vi "Actor Core Dups.vi"(8 "error in":errorcluster, 11 "Stepper3D in":refnum<class "Stepper3D.lvclass">) -> (0 "error out":errorcluster, 3 "Actor  out":refnum<class "Actor.lvclass">)   [LabVIEW 2014]
uses:
  <vilib>/Utility/config.llb/NI_LVConfig.lvlib
  <vilib>/Utility/error.llb/DialogType.ctl
  Libs/array.lib/Array.lvlib
  Libs/stepper3D.lib/stepper3D.lvlib
  Libs/stepper3D.lib/Enums/BoundaryStatus.ctl
  <vilib>/Utility/config.llb/Read Key (Double).vi
  <vilib>/Utility/config.llb/Write Key (Double).vi
  Framework/Interfaces/Viewable Actor/Viewable Actor.lvclass
  Framework/Interfaces/Observable Actor/Observable Actor.lvclass
  Framework/Model/Data/DataSingleElement/DataSingleElement.lvclass
  Framework/Hardware/ParameterDevice/ParameterDevice Messages/Set Parameter Msg/Set Parameter Msg.lvclass
  <vilib>/ActorFramework/Actor/Actor.lvclass
  Stepper3D Messages/Set Conversion Table Msg/Set Conversion Table Msg.lvclass
  Libs/stepper3D.lib/Enums/CurrentStatus.ctl
  Stepper3D Messages/Refresh Info Msg/Refresh Info Msg.lvclass
  Framework/Hardware/Device/Device Messages/Connect Msg/Connect Msg.lvclass
  Framework/Hardware/Device/Device Messages/Disconnect Msg/Disconnect Msg.lvclass
  Stepper3D.lvclass
panel:
  out "WL:Real Value":dbl=450.0
  out "Stop":bool=TRUE
  out "St3:Right":bool
  out "St3:Left":bool
  out "St2:Right":bool
  out "St2:Left":bool
  out "St1:Right":bool
  out "St1:Left":bool
  in  "Speed":string="300"
  in  "UI:LoadConversionTables":bool
  in  "Conversion 3":path=path "C:/Users/219-PC/Dropbox/МФД/Alexandr Bogomolov/Кумарин 47/Эталон.txt"
  in  "Conversion 2":path=path "C:/Users/219-PC/Dropbox/МФД/Alexandr Bogomolov/Кумарин 47/Эталон.txt"
  in  "Conversion 1":path=path "C:/Users/219-PC/Dropbox/МФД/Alexandr Bogomolov/Кумарин 47/Решетка 3D.txt"
  out "WL:WLToStepper3":dbl[][](array[numeric])
  out "WL:WLToStepper2":dbl[][](array[numeric])=[[115.0, 0.0], [135.0, 0.0]]
  out "WL:WLToStepper1":dbl[][](array[numeric])
  in  "WL:NewValue":dbl=450.0
  in  "WL:Stop":bool
  in  "WL:SetValue":bool
  out "App:RefreshLED":bool
  in  "App:RefreshRate":u32=500 caption="Refresh every"
  in  "App:Refresh":bool
  in  "App:Disconnect":bool
  in  "App:Connect":bool
  in  "St3:SetPos":bool
  in  "St2:SetPos":bool
  in  "St1:SetPos":bool
  in  "St:Stop":bool
  in  "St3:Steps":dbl
  in  "St3:NewPosition":dbl=2605.0
  out "St3:Position":dbl=2903.0
  in  "St2:Steps":dbl
  in  "St2:NewPosition":dbl=-2500.0
  out "St2:Position":dbl=-2500.0
  in  "St:DoSteps":bool
  in  "St1:Steps":dbl
  in  "St1:NewPosition":dbl=-57680.0
  out "St1:Position":dbl=-57680.0
  in  "App:ResourceName":refnum<visa-resource-name>="COM8"
  # "ms."
  # "BOUNDARY"
  # "FUNCTIONS"
  # "POSITION"
  # "NEW POSITION"
  # "STEPS"
  # "Решетка"
  # "Фабри-Перо"
  # "Кристалл"
  # "Длина волны"
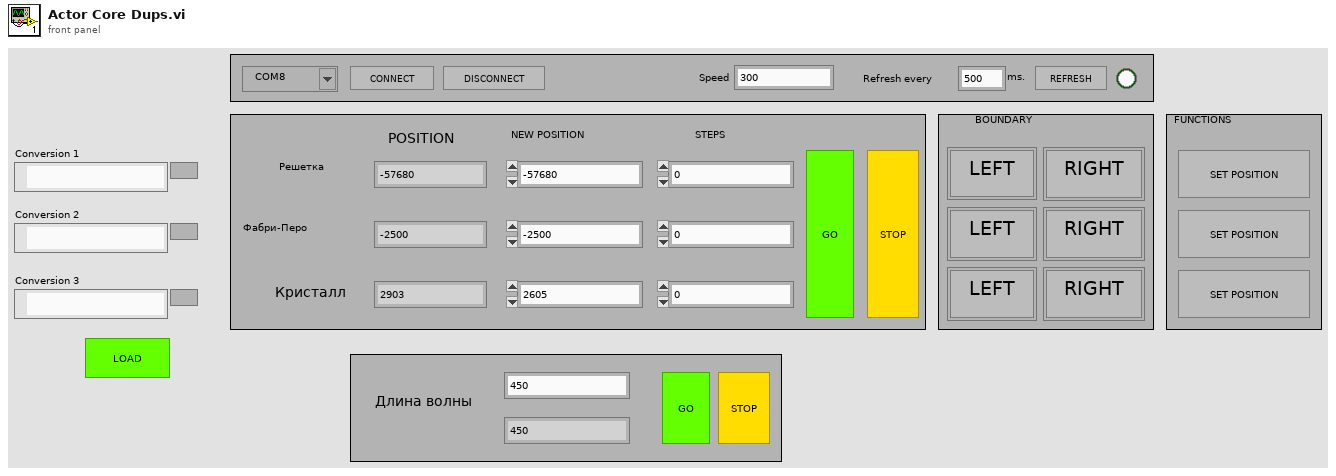
[diagram p1: front panel]
types:
  T1 = typedef "Observable Actor.lvlib/Observable Actor.lvclass/Observer.ctl" = refnum<queue>
  T2 = typedef "stepper3D.lvlib/CurrentStatus.ctl" = cluster{"desired":dbl[], "current":dbl[], "boundaries":T3[], "is running":bool}
  T3 = typedef "stepper3D.lvlib/BoundaryStatus.ctl" = enum16{"NO BOUNDARY", "OUT OF LEFT", "OUT OF RIGHT"}
  T4 = enum32{"invalid app kind", "Development System", "Run Time System", "Student Edition", "Embedded LabVIEW", "Evaluation", "Custom"}
  T5 = cluster{"Core":cluster{"Current VI Reference":refnum<vi>, "Close Panel on Exit?":bool}, "App:RefreshRate":u32, "appended path":path, "App:ResourceName":refnum<visa-resource-name>}
  T6 = typedef "DialogType.ctl" = u16
  T7 = cluster{"Current VI Reference":refnum<vi>, "Close Panel on Exit?":bool}
  T8 = typedef "NI_LVConfig.lvlib/Config Data RefNum.ctl" = refnum<k1>
  T9 = enum8{"Enabled", "Disabled", "Disabled and Grayed Out"}
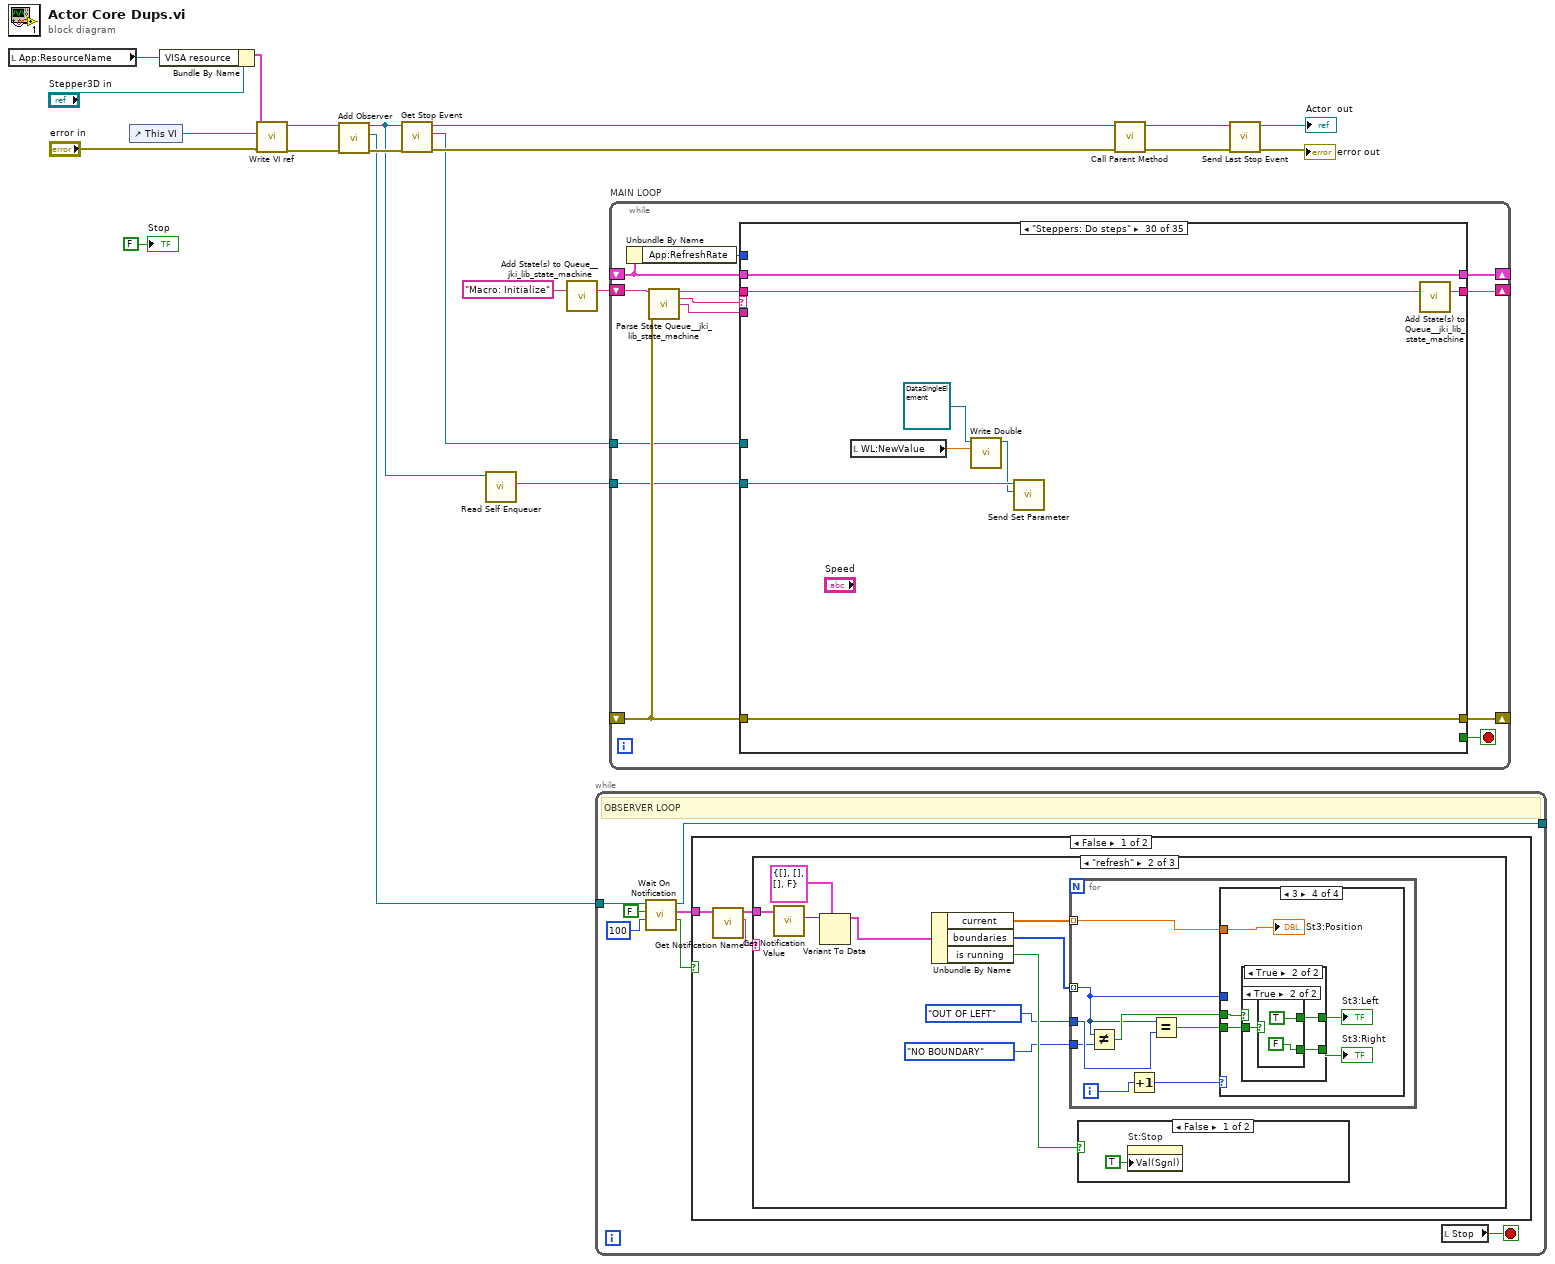
[diagram p0: block diagram]
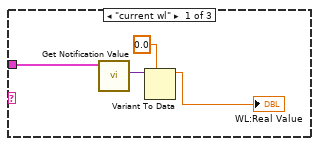
[diagram p2: hidden frame]
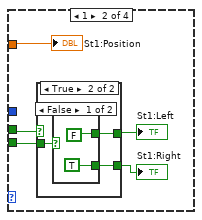
[diagram p5: hidden frame]
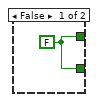
[diagram p6: hidden frame]
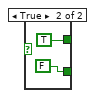
[diagram p7: hidden frame]
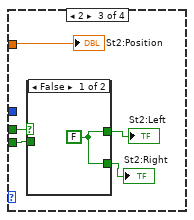
[diagram p8: hidden frame]
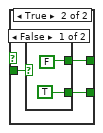
[diagram p9: hidden frame]
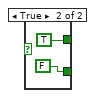
[diagram p10: hidden frame]
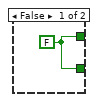
[diagram p11: hidden frame]
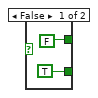
[diagram p12: hidden frame]
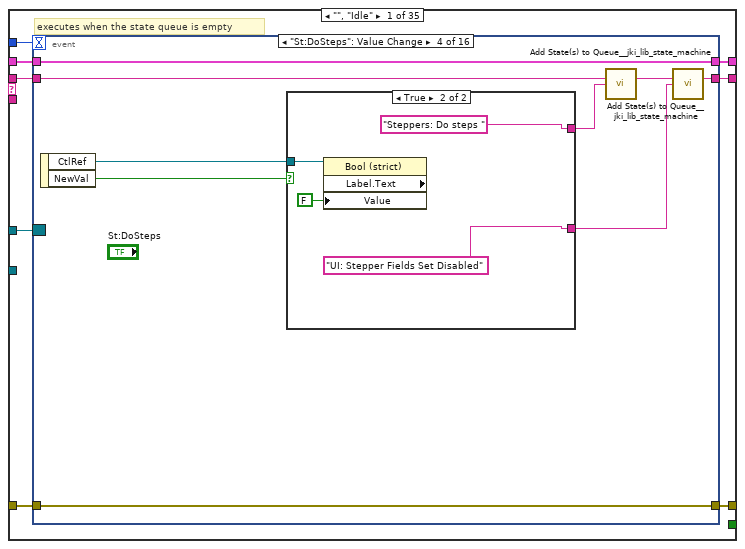
[diagram p15: hidden frame]
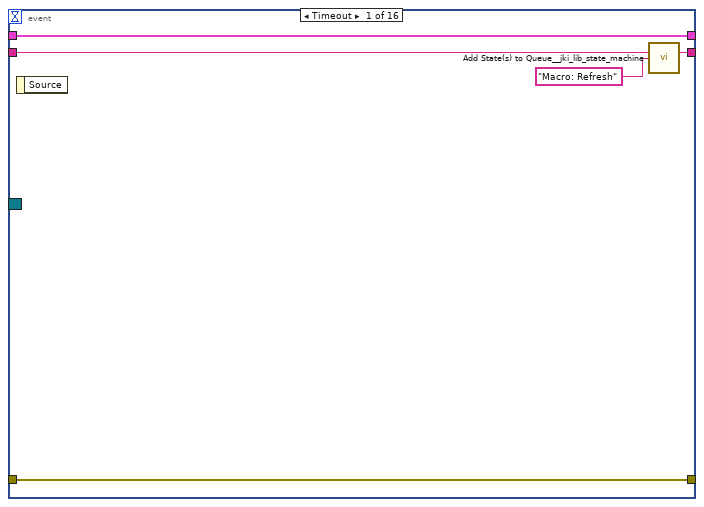
[diagram p16: hidden frame]
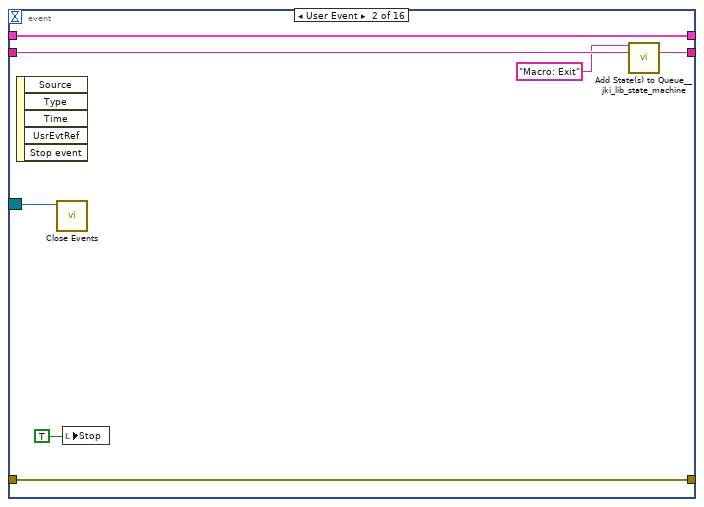
[diagram p17: hidden frame]
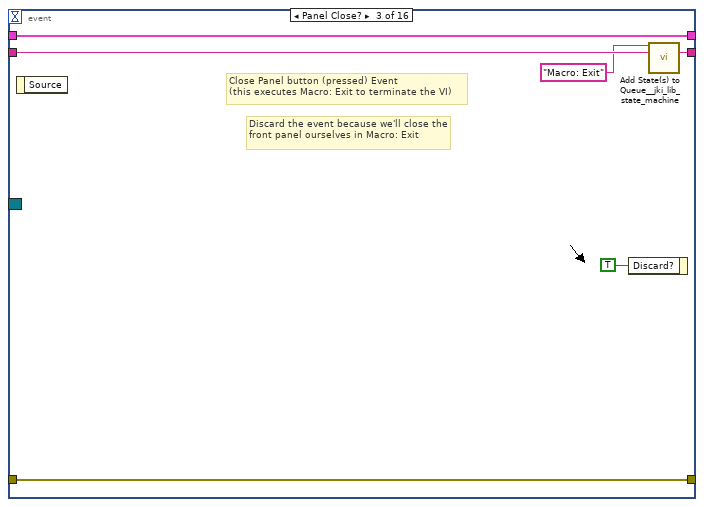
[diagram p18: hidden frame]
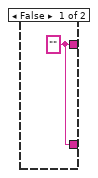
[diagram p19: hidden frame]
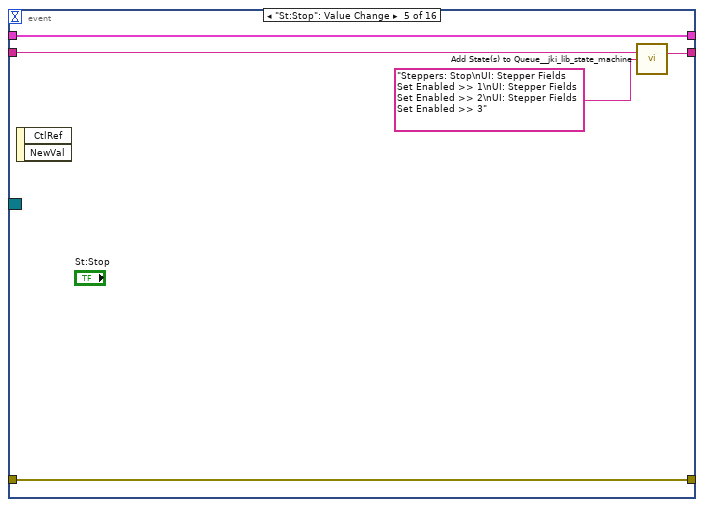
[diagram p20: hidden frame]
diagram:
  n1 = local read "App:ResourceName"() -> (w1:refnum<visa-resource-name>)
  n2 = control-ref of="This VI"() -> (w16:refnum<vi>)
  n3 = Bundle By Name(cluster="Stepper3D in", "VISA resource"=w1) -> (w3:cluster{})
  n4 = call "Write VI ref.vi"("error in (no error)"="error in", "VI ref"=w16, "Viewable Actor in"=w3) -> ("error out"=w18:errorcluster, "Viewable Actor out"=w17:refnum<class "Viewable Actor.lvclass">)  [unwired: 7 in]
  n5 = call-dynamic "Add Observer.vi"("error in (no error)"=w18, "Observable Actor in"=w17) -> ("error out"=w19:errorcluster, "new observer"=w6:T1, "Observable Actor out"=w5:refnum<class "Viewable Actor.lvclass">)  [unwired: 7 in]
  n6 = call-dynamic "Get Stop Event.vi"("error in (no error)"=w19, "Observable Actor in"=w5) -> ("error out"=w10:errorcluster, "Events"=w7:refnum<event-registration>, "Observable Actor out"=w11:refnum<class "Viewable Actor.lvclass">)  [unwired: 7 in]
  n7 = call <vilib>:"Read Self Enqueuer.vi"("Actor"=w5) -> ("Self Enqueuer"=w4:refnum<class "Message Enqueuer.lvclass">)  [unwired: 10 in]
  n8 = call <vilib>:"Add State(s) to Queue__jki_lib_state_machine.vi"("State(s) in (\"\")"="Macro: Initialize") -> ("States Out"=w21:string)  [unwired: 14 in]
  n9 = while {
    tunnel: w6 -> [w26]
    tunnel: [w25] -> _
    stop <- w22 stop-if-true
    # "OBSERVER LOOP"
    n10 = call "Wait On Notification.vi"("timeout in ms (-1)"=100, "ignore previous (F)"=FALSE, "observer in"=w26) -> ("timed out?"=w23:bool, "notification"=w24:cluster{"value":variant, "name":string}, "observer out"=w25:T1)  [unwired: 5 in, 1 out]
    n11 = case shown="False" w23 {
      tunnel: w24 -> [w31 _]
      frame False {
        n12 = call "Get Notification Name.vi"("notification in"=w31) -> ("name"=w29:string, "notification out"=w30:cluster{"value":variant, "name":string})  [unwired: 9 in]
        n13 = case shown="\"refresh\"" w29 {
          tunnel: w30 -> [w33 w43 _]
          frame "current wl" {
            n14 = call "Get Notification Value.vi"("notification in"=w33) -> ("data"=w35:variant)  [unwired: 7 in, 1 out]
            n15 = Variant To Data(type=0.0 ("Current value"), Variant=w35) -> (data=→"WL:Real Value":dbl)  [unwired: 1 in, 1 out]
          }
          frame "refresh" {
            n16 = call "Get Notification Value.vi"("notification in"=w43) -> ("data"=w44:variant)  [unwired: 7 in, 1 out]
            n17 = Variant To Data(type=T2 {"desired"=[], "current"=[], "boundaries"=[], "is running"=FALSE} ("status"), Variant=w44) -> (data=w37:T2)  [unwired: 1 in, 1 out]
            n18 = Unbundle By Name(w37) -> ("current"=w38:dbl[], "boundaries"=w39:T3[], "is running"=w42:bool)
            n19 = for {
              tunnel: w38 -> [w51] mode=indexing
              tunnel: w39 -> [w48] mode=indexing
              tunnel: BoundaryStatus."NO BOUNDARY" ("Enum") -> [w46]
              tunnel: BoundaryStatus."OUT OF LEFT" ("Enum") -> [w49]
              i -> [w53]
              n20 = Not Equal?(x=w48, y=w46) -> (x != y?=w50:bool)
              n21 = Increment(x=w53) -> (x+1=w52:i32)
              n22 = Equal?(x=w48, y=w49) -> (x = y?=w47:bool)
              n23 = case shown="3" w52 {
                tunnel: w51 -> [_ w58 w71 w84]
                tunnel: w48 -> [_ _ _ _]
                tunnel: w50 -> [_ w57 w70 w83]
                tunnel: w47 -> [_ w56 w69 w82]
                frame Default {
                }
                frame 1 {
                  n24 = case shown="True" w57 {
                    tunnel: w56 -> [_ w62]
                    tunnel: [w59 w61] -> w55
                    tunnel: [w59 w60] -> w54
                    frame False {
                      w59 = FALSE
                    }
                    frame True {
                      n25 = case shown="False" w62 {
                        tunnel: [FALSE TRUE] -> w61
                        tunnel: [TRUE FALSE] -> w60
                        frame False {
                        }
                        frame True {
                        }
                      }
                    }
                  }
                  "St1:Right" <- w54
                  "St1:Left" <- w55
                  "St1:Position" <- w58
                }
                frame 2 {
                  n26 = case shown="False" w70 {
                    tunnel: w69 -> [_ w75]
                    tunnel: [w72 w74] -> w68
                    tunnel: [w72 w73] -> w67
                    frame False {
                      w72 = FALSE
                    }
                    frame True {
                      n27 = case shown="False" w75 {
                        tunnel: [FALSE TRUE] -> w74
                        tunnel: [TRUE FALSE] -> w73
                        frame False {
                        }
                        frame True {
                        }
                      }
                    }
                  }
                  "St2:Left" <- w68
                  "St2:Right" <- w67
                  "St2:Position" <- w71
                }
                frame 3 {
                  n28 = case shown="True" w83 {
                    tunnel: w82 -> [_ w88]
                    tunnel: [w85 w87] -> w80
                    tunnel: [w85 w86] -> w81
                    frame False {
                      w85 = FALSE
                    }
                    frame True {
                      n29 = case shown="True" w88 {
                        tunnel: [FALSE TRUE] -> w87
                        tunnel: [TRUE FALSE] -> w86
                        frame False {
                        }
                        frame True {
                        }
                      }
                    }
                  }
                  "St3:Left" <- w80
                  "St3:Right" <- w81
                  "St3:Position" <- w84
                }
              }
            }
            n30 = case shown="False" w42 {
              frame False {
                n31 = property on="St:Stop" class="Bool (strict)"("Val(Sgnl)"=TRUE) -> ()  [unwired: 2 in, 2 out]
              }
              frame True {
              }
            }
          }
          frame Default {
          }
        }
      }
      frame True {
      }
    }
    n32 = local read "Stop"() -> (w22:bool)
  }
  n33 = while "MAIN LOOP" {
    shift-right: [w99] -> _
    shift-left: _ -> [w95]
    shift-right: [w102] -> _
    shift-left: _ -> [w98]
    shift-right: [w101] -> _
    shift-left: w21 -> [w103]
    tunnel: w7 -> [w94]
    tunnel: w4 -> [w93]
    stop <- w100 stop-if-true
    n34 = Unbundle By Name(w95) -> ("App:RefreshRate"=w96:u32)
    n35 = call <vilib>:"Parse State Queue__jki_lib_state_machine.vi"("State Queue"=w103, "Error In (no error)"=w98) -> ("Remaining States"=w105:string, "Current State"=w97:string, "Arguments"=w104:string)  [unwired: 11 in]
    n36 = case shown="\"Steppers: Do steps\"" w97 {
      selector: w97 -> [_ _ w260 _ _ _ _ _ _ _ _ _ _ _ _ _ _ _ _ _ _ _ _ _ _ _ _ _ _ _ _ _ _ _ _]
      tunnel: w105 -> [w113 w259 w264 w282 w289 w294 w298 w315 w325 w344 w366 w372 w376 w381 w386 w391 w393 w412 w415 w431 w432 w439 w454 w459 w464 w474 w478 w484 w490 w498 w513 w524 w530 w535 w542]
      tunnel: w104 -> [_ _ _ _ _ _ _ _ _ _ _ _ _ _ _ _ w392 _ w416 _ w435 w440 _ _ _ _ _ _ _ _ w509 _ _ _ w538]
      tunnel: w95 -> [w111 w256 w262 w273 w286 w292 w295 w312 _ w342 w363 w368 w373 w378 w383 w389 w395 w414 w418 w429 w436 w442 w451 w456 w461 w471 w475 w480 w486 w496 w510 w522 w531 w532 w539]
      tunnel: [w110 w257 w266 w279 errorcluster {"status"=FALSE, "code"=0, "source"=""} ("error out") w291 w296 w313 w322 w326 w364 w369 w374 w379 w384 w388 w394 w413 w417 w428 w434 w443 w452 w457 w462 w472 w476 w479 w487 w495 w508 w519 w525 w533 w540] -> w102
      tunnel: w98 -> [w109 w257 w265 w279 w285 w291 w296 w313 w322 w327 w364 w367 w374 w379 w384 w388 w394 w413 w417 w428 w434 w444 w452 w457 w462 w472 w476 w481 w488 w495 w507 w520 w526 w533 w540]
      tunnel: [w112 w258 w263 w281 w288 w293 w297 w314 w324 w343 w365 w371 w375 w380 w385 w390 w393 w412 w415 w430 w432 w439 w453 w458 w463 w473 w477 w485 w490 w497 w512 w523 w529 w534 w541] -> w101
      tunnel: [_ _ _ _ _ TRUE _ _ _ _ _ _ _ _ _ _ _ _ _ _ _ _ _ _ _ _ _ _ _ _ _ _ _ _ _] -> w100
      tunnel: [w108 w256 w262 w280 w286 w292 w295 w312 w323 w342 w363 w368 w373 w378 w383 w389 w395 w414 w418 w429 w436 w442 w451 w456 w461 w471 w475 w480 w486 w496 w510 w522 w531 w532 w539] -> w99
      tunnel: w96 -> [w107 _ _ _ _ _ _ _ _ _ _ _ _ _ _ _ _ _ _ _ _ _ _ _ _ _ _ _ _ _ _ _ _ _ _]
      tunnel: w94 -> [w106 _ _ _ _ _ _ _ _ _ _ _ _ _ _ _ _ _ _ _ _ _ _ _ _ _ _ _ _ _ _ _ _ _ _]
      tunnel: w93 -> [_ _ _ _ _ _ _ w305 _ _ _ _ _ _ _ _ _ _ _ _ _ _ _ _ _ _ _ w482 w489 w494 _ _ w527 _ _]
      frame "", "Idle" {
        # "executes when the state queue is empty"
        n37 = event shown="[3] \"St:DoSteps\": Value Change" {
          selector: w106 -> [_ w121 _ _ _ _ _ _ _ _ _ _ _ _ _ _]
          dyn-events: _ -> [_ _ _ _ _ _ _ _ _ _ _ _ _ _ _ _]
          timeout: w107 -> [_ _ _ _ _ _ _ _ _ _ _ _ _ _ _ _]
          tunnel: w113 -> [w118 w122 w131 w136 w147 w153 w174 w185 w192 w202 w213 w227 w232 w237 w244 w252]
          tunnel: [w117 w123 w130 w134 w148 w152 w173 w184 w193 w203 w214 w228 w233 w238 w245 w253] -> w112
          tunnel: w111 -> [w115 w124 w128 w139 w150 w156 w176 w187 w194 w206 w217 w224 w230 w235 w242 w250]
          tunnel: [w116 w119 w129 w138 w149 w155 w175 w186 w195 w200 w211 w225 w231 w236 w243 w251] -> w110
          tunnel: w109 -> [w116 w119 w129 w138 w149 w155 w175 w186 w195 w200 w211 w225 w231 w236 w243 w251]
          tunnel: [w115 w124 w128 w139 w150 w156 w176 w187 w194 w206 w217 w223 w230 w235 w242 w250] -> w108
          event Timeout {
            n38 = event-data() -> ()  [unwired: 1 in, 1 out]
            n39 = call <vilib>:"Add State(s) to Queue__jki_lib_state_machine.vi"("State(s) in (\"\")"=w118, "State(s) at Back (\"\")"="Macro: Refresh") -> ("States Out"=w117:string)  [unwired: 13 in]
          }
          event User Event {
            n40 = event-data() -> ()  [unwired: 1 in, 5 out]
            n41 = call "Close Events.vi"("events"=w121) -> ()  [unwired: 11 in]
            n42 = local write "Stop"(TRUE) -> ()
            n43 = call <vilib>:"Add State(s) to Queue__jki_lib_state_machine.vi"("State(s) in Front (\"\")"="Macro: Exit", "State(s) in (\"\")"=w122) -> ("States Out"=w123:string)  [unwired: 13 in]
          }
          event Panel Close? {
            # "Discard the event because we'll close the front panel ourselves in Macro: Exit"
            # "Close Panel button (pressed) Event\n(this executes Macro: Exit to terminate the VI)"
            n44 = event-data() -> ()  [unwired: 1 in, 1 out]
            n45 = event-data("Discard?"=TRUE) -> ()  [unwired: 1 in, 1 out]
            n46 = call <vilib>:"Add State(s) to Queue__jki_lib_state_machine.vi"("State(s) in Front (\"\")"="Macro: Exit", "State(s) in (\"\")"=w131) -> ("States Out"=w130:string)  [unwired: 13 in]
          }
          event "St:DoSteps": Value Change {
            n47 = event-data() -> ("CtlRef"=w140:refnum<vi>, "NewVal"=w137:bool)  [unwired: 1 in]
            n48 = case shown="True" w137 {
              tunnel: w140 -> [_ w145]
              tunnel: [w141 "Steppers: Do steps "] -> w135
              tunnel: [w141 "UI: Stepper Fields Set Disabled" ("State")] -> w132
              frame False {
                w141 = "" ("State with Arguments")
              }
              frame True {
                n49 = property class="Bool (strict)" props=["Label", "Text", "Value"](reference=w145, "Value"=FALSE) -> ()  [unwired: 1 in, 3 out]
              }
            }
            n50 = call <vilib>:"Add State(s) to Queue__jki_lib_state_machine.vi"("State(s) in (\"\")"=w136, "State(s) at Back (\"\")"=w135) -> ("States Out"=w133:string)  [unwired: 13 in]
            n51 = call <vilib>:"Add State(s) to Queue__jki_lib_state_machine.vi"("State(s) in (\"\")"=w133, "State(s) at Back (\"\")"=w132) -> ("States Out"=w134:string)  [unwired: 13 in]
          }
          event "St:Stop": Value Change {
            n52 = event-data() -> ()  [unwired: 1 in, 2 out]
            n53 = call <vilib>:"Add State(s) to Queue__jki_lib_state_machine.vi"("State(s) in (\"\")"=w147, "State(s) at Back (\"\")"="Steppers: Stop\nUI: Stepper Fields Set Enabled >> 1\nUI: Stepper Fields Set Enabled >> 2\nUI: Stepper Fields Set Enabled >> 3" ("State")) -> ("States Out"=w148:string)  [unwired: 13 in]
          }
          event "St1:SetPos", "St2:SetPos", "St3:SetPos": Value Change {
            n54 = event-data() -> ("CtlRef"=w157:refnum<vi>, "NewVal"=w154:bool)  [unwired: 1 in]
            n55 = case shown="True" w154 {
              tunnel: w157 -> [_ w166]
              tunnel: ["" ("State with Arguments") w160] -> w151
              frame False {
              }
              frame True {
                n56 = property class="Bool (strict)"(reference=w166, "Value"=FALSE) -> ("Label.Text"=w163:string)  [unwired: 1 in, 2 out]
                n57 = String Subset(string=w163, offset (0)=2, length (rest)=1 ("length (rest)")) -> (substring=w161:string)
                n58 = call <vilib>:"Build State String with Arguments__jki_lib_state_machine.vi"("Arguments (\"\")"=w161, "State"="Steppers: Set position") -> ("State with Arguments"=w160:string)  [unwired: 4 in]
              }
            }
            n59 = call <vilib>:"Add State(s) to Queue__jki_lib_state_machine.vi"("State(s) in (\"\")"=w153, "State(s) at Back (\"\")"=w151) -> ("States Out"=w152:string)  [unwired: 13 in]
          }
          event "St1:NewPosition", "St2:NewPosition", "St3:NewPosition": Value Change {
            n60 = event-data() -> ("CtlRef"=w177:refnum<vi>)  [unwired: 1 in]
            n61 = property class="DigNum (strict)"(reference=w177) -> ("Label.Text"=w169:string)  [unwired: 1 in, 2 out]
            n62 = String Subset(string=w169, offset (0)=2, length (rest)=1 ("length (rest)")) -> (substring=w167:string)
            n63 = call <vilib>:"Build State String with Arguments__jki_lib_state_machine.vi"("Arguments (\"\")"=w167, "State"="UI: New position to steps") -> ("State with Arguments"=w172:string)  [unwired: 4 in]
            n64 = call <vilib>:"Add State(s) to Queue__jki_lib_state_machine.vi"("State(s) in (\"\")"=w174, "State(s) at Back (\"\")"=w172) -> ("States Out"=w173:string)  [unwired: 13 in]
          }
          event "St1:Steps", "St2:Steps", "St3:Steps": Value Change {
            n65 = event-data() -> ("CtlRef"=w188:refnum<vi>)  [unwired: 1 in]
            n66 = property class="DigNum (strict)"(reference=w188) -> ("Label.Text"=w180:string)  [unwired: 1 in, 2 out]
            n67 = String Subset(string=w180, offset (0)=2, length (rest)=1 ("length (rest)")) -> (substring=w178:string)
            n68 = call <vilib>:"Build State String with Arguments__jki_lib_state_machine.vi"("Arguments (\"\")"=w178, "State"="UI: Steps to new position") -> ("State with Arguments"=w183:string)  [unwired: 4 in]
            n69 = call <vilib>:"Add State(s) to Queue__jki_lib_state_machine.vi"("State(s) in (\"\")"=w185, "State(s) at Back (\"\")"=w183) -> ("States Out"=w184:string)  [unwired: 13 in]
          }
          event "App:Connect": Value Change {
            n70 = event-data() -> ("CtlRef"=w191:refnum<vi>, "NewVal"=w190:bool)  [unwired: 1 in]
            n71 = case shown="True" w190 {
              tunnel: w191 -> [_ w199]
              tunnel: ["" "UI: Cursor Set >> Busy\nSteppers: Connect\nUtils: Wait ms >> 1000\nUI: Cursor Set >> Idle"] -> w189
              frame False {
              }
              frame True {
                n72 = property class="Bool (strict)"(reference=w199, "Value"=FALSE) -> ()  [unwired: 1 in, 2 out]
              }
            }
            n73 = call <vilib>:"Add State(s) to Queue__jki_lib_state_machine.vi"("State(s) in (\"\")"=w192, "State(s) at Back (\"\")"=w189) -> ("States Out"=w193:string)  [unwired: 13 in]
          }
          event "App:Disconnect": Value Change {
            n74 = event-data() -> ("CtlRef"=w205:refnum<vi>, "NewVal"=w204:bool)  [unwired: 1 in]
            n75 = case shown="True" w204 {
              tunnel: w205 -> [_ w210]
              tunnel: ["" "Steppers: Disconnect"] -> w201
              frame False {
              }
              frame True {
                n76 = property class="Bool (strict)"(reference=w210, "Value"=FALSE) -> ()  [unwired: 1 in, 2 out]
              }
            }
            n77 = call <vilib>:"Add State(s) to Queue__jki_lib_state_machine.vi"("State(s) in (\"\")"=w202, "State(s) at Back (\"\")"=w201) -> ("States Out"=w203:string)  [unwired: 13 in]
          }
          event "App:Refresh": Value Change {
            n78 = event-data() -> ("CtlRef"=w216:refnum<vi>, "NewVal"=w215:bool)  [unwired: 1 in]
            n79 = case shown="True" w215 {
              tunnel: w216 -> [_ w221]
              tunnel: ["" "Macro: Refresh"] -> w212
              frame False {
              }
              frame True {
                n80 = property class="Bool (strict)"(reference=w221, "Value"=FALSE) -> ()  [unwired: 1 in, 2 out]
              }
            }
            n81 = call <vilib>:"Add State(s) to Queue__jki_lib_state_machine.vi"("State(s) in (\"\")"=w213, "State(s) at Back (\"\")"=w212) -> ("States Out"=w214:string)  [unwired: 13 in]
          }
          event "App:RefreshRate": Value Change {
            n82 = event-data() -> ()  [unwired: 1 in, 1 out]
            n83 = Bundle By Name(cluster=w224, "App:RefreshRate"="App:RefreshRate") -> (w223:T5)
            n84 = call <vilib>:"Add State(s) to Queue__jki_lib_state_machine.vi"("State(s) in (\"\")"=w227, "State(s) at Back (\"\")"="Steppers: Set refresh rate") -> ("States Out"=w228:string)  [unwired: 13 in]
          }
          event "WL:NewValue": Value Change {
            n85 = event-data() -> ()  [unwired: 1 in, 6 out]
            n86 = call <vilib>:"Add State(s) to Queue__jki_lib_state_machine.vi"("State(s) in (\"\")"=w232, "State(s) at Back (\"\")"="UI: New WL to positions" ("State(s) at Back (\"\")")) -> ("States Out"=w233:string)  [unwired: 13 in]
          }
          event "WL:SetValue": Value Change {
            n87 = event-data() -> ("NewVal"=w234:bool)  [unwired: 1 in]
            n88 = case shown="True" w234 {
              frame False {
              }
              frame True {
                n89 = property on="WL:SetValue" class="Bool (strict)"("Value"=FALSE ("WL:SetValue")) -> ()  [unwired: 2 in, 2 out]
                n90 = property on="St:DoSteps" class="Bool (strict)"("Val(Sgnl)"=TRUE) -> ()  [unwired: 2 in, 2 out]
              }
            }
            n91 = call <vilib>:"Add State(s) to Queue__jki_lib_state_machine.vi"("State(s) in (\"\")"=w237) -> ("States Out"=w238:string)  [unwired: 14 in]
          }
          event "WL:Stop": Value Change {
            n92 = event-data() -> ("NewVal"=w241:bool)  [unwired: 1 in]
            n93 = case shown="True" w241 {
              frame False {
              }
              frame True {
                n94 = property on="WL:Stop" class="Bool (strict)"("Value"=FALSE ("WL:Stop")) -> ()  [unwired: 2 in, 2 out]
                n95 = property on="St:Stop" class="Bool (strict)"("Val(Sgnl)"=TRUE) -> ()  [unwired: 2 in, 2 out]
              }
            }
            n96 = call <vilib>:"Add State(s) to Queue__jki_lib_state_machine.vi"("State(s) in (\"\")"=w244) -> ("States Out"=w245:string)  [unwired: 14 in]
          }
          event "UI:LoadConversionTables": Value Change {
            n97 = event-data() -> ("NewVal"=w249:bool)  [unwired: 1 in]
            n98 = case shown="True" w249 {
              tunnel: [_ "Data: Load Conversion Files"] -> w248
              frame False {
              }
              frame True {
                n99 = property on="UI:LoadConversionTables" class="Bool (strict)"("Value"=FALSE) -> ()  [unwired: 2 in, 2 out]
              }
            }
            n100 = call <vilib>:"Add State(s) to Queue__jki_lib_state_machine.vi"("State(s) in (\"\")"=w252, "State(s) at Back (\"\")"=w248) -> ("States Out"=w253:string)  [unwired: 13 in]
          }
        }
      }
      frame "---------- Core ----------" {
        # "Do not put any code in this frame.\n(it is a separator no-op)"
        n101 = call <vilib>:"Add State(s) to Queue__jki_lib_state_machine.vi"("State(s) in (\"\")"=w259) -> ("States Out"=w258:string)  [unwired: 14 in]
      }
      frame Default {
        w269 = 42 items=["No error", "Argument error", "Memory is full", "Out of zone", "End of file", "File already open", "Generic file I/O error", "File not found", "File permission error", "Disk is full", "Duplicate path", "Too many files open", "System feature not enabled", "Resource file not found", "Cannot add resource", "Resource not found", "Image not found", "Image memory error", "Pen does not exist", "Config type invalid", "Config token not found", "Config parse error", "Config memory error", "Bad external code format", "Bad external code offset", "External code not present", "Null window", "Destroy window error", "Null menu", "Print aborted", "Bad print record", "Print driver error", "Windows error during printing", "Memory error during printing", "Print dialog error", "Generic print error", "Invalid device refnum", "Device not found", "Device parameter error", "Device unit error", "Cannot open device", "Device call aborted", "Generic error", "Cancelled by user", "Object ID too low", "Object ID too high", "Object not in heap", "Unknown heap", "Unknown object (invalid DefProc)", "Unknown object (DefProc not in table)", "Message out of range", "Invalid (null) method", "Unknown message", "Manager call not supported", "Bad address", "Network operation in progress", "Network operation timed out", "Connection is busy", "Network attribute not supported", "Network error", "Address in use", "System out of memory", "Connection aborted", "Connection refused", "Not connected", "Already connected", "Connection closed", "Initialization error (interapplication manager)", "Bad occurrence", "Wait on unbound occurrence handler", "Occurrence queue overflow", "Datalog type conflict", "Unused", "Unrecognized type (interapplication manager)", "Memory corrupt", "Failed to make temporary DLL", "Old CIN version", "Drag socket not found", "Failed to load drop-object", "Failed to register OLE object", "Failed to release OLE object", "Format specifier type mismatch", "Unknown format specifier", "Too few format specifiers", "Too many format specifiers", "Scan failed", "Newer CIN version", "Error converting to variant", "Runtime menu error", "Password tampered", "Variant attribute not found", "Incompatible variant data type", "Event data is not available", "Event Store is not present", "Occurrence is not found", "Event Queue is not created", "Event info is not available", "Refnum passed is NULL", "Error retrieving Class GUID", "Error retrieving CoClass GUID", "Error retrieving TypeLib GUID.", "Bad built application magic bytes.", "Specific driver is different from the specific driver associated with the Logical Name.", "There is no session opened to the class driver.", "Max Error", "MAX - Error with config objects", "MAX - Error loading configuration", "MAX - Group not supported"]
        # "Current State"
        # "Handle mistyped state name (developer tool)"
        n102 = Format Into String(format string="Software Exception: Unhandled State \"%s\"." ("message"), error in=w265, w260) -> (resulting string=w268:string, error out=w267:errorcluster)  [unwired: 1 in]
        n103 = call <vilib>:"Error Cluster From Error Code.vi"("show call chain? (False)"=TRUE, "error in (no error)"=w267, "error message (\"\")"=w268, "error code (0)"=w269) -> ("error out"=w266:errorcluster)  [unwired: 5 in]
        n104 = call <vilib>:"Add State(s) to Queue__jki_lib_state_machine.vi"("State(s) in (\"\")"=w264) -> ("States Out"=w263:string)  [unwired: 14 in]
      }
      frame "Initialize Core Data" {
        # "originally closed?"
        # "exe?"
        # "If panel starts closed or is an EXE, then close it when we exit"
        n105 = property class="VI"() -> ("Front Panel.Open"=w278:bool)  [unwired: 2 in, 2 out]
        n106 = property class="App"() -> ("App.Kind"=w277:T4)  [unwired: 2 in, 2 out]
        n107 = control-ref of="Current VI Reference"() -> (w271:refnum<vi>)
        n108 = Not(x=w278) -> (.not. x?=w275:bool)
        n109 = Equal?(x=w277, y=T4."Run Time System" ("Application:Kind")) -> (x = y?=w274:bool)
        n110 = Or(x=w275, y=w274) -> (x .or. y?=w272:bool)
        n111 = Bundle By Name(cluster=w273, "Core.Current VI Reference"=w271, "Core.Close Panel on Exit?"=w272) -> (w280:T5)
        n112 = call <vilib>:"Add State(s) to Queue__jki_lib_state_machine.vi"("State(s) in (\"\")"=w282) -> ("States Out"=w281:string)  [unwired: 14 in]
      }
      frame "Error Handler" {
        w283 = T6 2 items=["no dialog", "OK message", "continue or stop message", "OK message + warnings", "continue/stop + warnings"] ("type of dialog (OK msg:1)")
        # "Unhandled Error -- Display it"
        # "Handle any errors here.\nYou can also output any states to clean-up after errors occur"
        # "Clear error"
        n113 = call <vilib>:"General Error Handler.vi"("type of dialog (OK msg:1)"=w283, "error in (no error)"=w285) -> ()  [unwired: 9 in, 5 out]
        n114 = call <vilib>:"Add State(s) to Queue__jki_lib_state_machine.vi"("State(s) in Front (\"\")"="// Post Error States", "State(s) in (\"\")"=w289) -> ("States Out"=w288:string)  [unwired: 13 in]
      }
      frame "Exit" {
        n115 = call <vilib>:"Add State(s) to Queue__jki_lib_state_machine.vi"("State(s) in (\"\")"=w294) -> ("States Out"=w293:string)  [unwired: 14 in]
      }
      frame "---------- Data ----------" {
        # "Do not put any code in this frame.\n(It is a separator no-op. You can make a copy of this frame to create a new Data frame)"
        n116 = call <vilib>:"Add State(s) to Queue__jki_lib_state_machine.vi"("State(s) in (\"\")"=w298) -> ("States Out"=w297:string)  [unwired: 14 in]
      }
      frame "Data: Load Conversion Files" {
        n117 = call "readArrayFromFile.vi"("file"="Conversion 1") -> ("array"=w307:dbl[][])  [unwired: 1 in, 1 out]
        "WL:WLToStepper1" <- w307
        n118 = call "readArrayFromFile.vi"("file"="Conversion 2") -> ("array"=w303:dbl[][])  [unwired: 1 in, 1 out]
        "WL:WLToStepper2" <- w303
        n119 = call "readArrayFromFile.vi"("file"="Conversion 3") -> ("array"=w299:dbl[][])  [unwired: 1 in, 1 out]
        "WL:WLToStepper3" <- w299
        n120 = call "Send Set Conversion Table.vi"("Stepper"=u32 1, "Conversion table"=w307, "Message Enqueuer"=w305) -> ("Message Enqueuer out"=w301:refnum<class "Message Enqueuer.lvclass">)  [unwired: 7 in, 1 out]
        n121 = call "Send Set Conversion Table.vi"("Stepper"=u32 2, "Conversion table"=w303, "Message Enqueuer"=w301) -> ("Message Enqueuer out"=w302:refnum<class "Message Enqueuer.lvclass">)  [unwired: 7 in, 1 out]
        n122 = call "Send Set Conversion Table.vi"("Stepper"=u32 3, "Conversion table"=w299, "Message Enqueuer"=w302) -> ()  [unwired: 7 in, 2 out]
        n123 = call <vilib>:"Add State(s) to Queue__jki_lib_state_machine.vi"("State(s) in (\"\")"=w315, "State(s) at Back (\"\")"="UI: New WL to positions" ("State(s) at Back (\"\")")) -> ("States Out"=w314:string)  [unwired: 13 in]
      }
      frame "Data: Initialize" {
        w321 = T7 {"Current VI Reference"=refnum, "Close Panel on Exit?"=FALSE}  # Core
        n124 = local read "App:RefreshRate"() -> (w320:u32)
        n125 = call <vilib>:"Application Directory.vi"() -> ("Application Directory"=w319:path)
        n126 = Build Path(base path=w319, name or relative path="steppers.config") -> (appended path=w317:path)
        n127 = Bundle("Core"=w321, "App:RefreshRate"=w320, "appended path"=w317, "App:ResourceName"="App:ResourceName") -> (w323:T5)  [unwired: 1 in]
        n128 = call <vilib>:"Add State(s) to Queue__jki_lib_state_machine.vi"("State(s) in (\"\")"=w325) -> ("States Out"=w324:string)  [unwired: 14 in]
      }
      frame "Data: Read Config" {
        n129 = Unbundle By Name(w342) -> ("appended path"=w329:path)
        n130 = call <vilib>:"Open Config Data.vi"("error in (no error)"=w327, "configuration file path"=w329) -> ("error out"=w326:errorcluster, "refnum"=w328:T8)  [unwired: 7 in, 1 out]
        n131 = call-poly <vilib>:"Read Key.vi"("section"="current values", "key"="wavelength", "refnum"=w328) -> ("value"=w333:dbl)  [unwired: 5 in, 3 out]
        n132 = call-poly <vilib>:"Read Key.vi"("section"="current values", "key"="stepper1", "refnum"=w328) -> ("value"=w332:dbl)  [unwired: 5 in, 3 out]
        n133 = call-poly <vilib>:"Read Key.vi"("section"="current values", "key"="stepper2", "refnum"=w328) -> ("value"=w331:dbl)  [unwired: 5 in, 3 out]
        n134 = call-poly <vilib>:"Read Key.vi"("section"="current values", "key"="stepper3", "refnum"=w328) -> ("value"=w330:dbl)  [unwired: 5 in, 3 out]
        n135 = local write "WL:NewValue"(w333) -> ()
        n136 = local write "St1:NewPosition"(w332) -> ()
        n137 = local write "St2:NewPosition"(w331) -> ()
        n138 = local write "St3:NewPosition"(w330) -> ()
        n139 = call <vilib>:"Add State(s) to Queue__jki_lib_state_machine.vi"("State(s) in (\"\")"=w344) -> ("States Out"=w343:string)  [unwired: 14 in]
      }
      frame "Data: Write Config" {
        n140 = Unbundle By Name(w363) -> ("appended path"=w347:path)
        n141 = local read "St1:Position"() -> (w353:dbl)
        n142 = local read "WL:NewValue"() -> (w354:dbl)
        n143 = local read "St2:Position"() -> (w352:dbl)
        n144 = local read "St3:Position"() -> (w351:dbl)
        n145 = call <vilib>:"Open Config Data.vi"("configuration file path"=w347) -> ("refnum"=w346:T8)  [unwired: 8 in, 2 out]
        n146 = call-poly <vilib>:"Write Key.vi"("section"="current values", "value"=w354, "key"="wavelength", "refnum"=w346) -> ("refnum out"=w350:T8)  [unwired: 5 in, 2 out]
        n147 = call-poly <vilib>:"Write Key.vi"("section"="current values", "value"=w353, "key"="stepper1", "refnum"=w350) -> ("refnum out"=w349:T8)  [unwired: 5 in, 2 out]
        n148 = call-poly <vilib>:"Write Key.vi"("section"="current values", "value"=w352, "key"="stepper2", "refnum"=w349) -> ("refnum out"=w348:T8)  [unwired: 5 in, 2 out]
        n149 = call-poly <vilib>:"Write Key.vi"("section"="current values", "value"=w351, "key"="stepper3", "refnum"=w348) -> ("refnum out"=w345:T8)  [unwired: 5 in, 2 out]
        n150 = call <vilib>:"Close Config Data.vi"("refnum"=w345) -> ()  [unwired: 9 in, 2 out]
        n151 = call <vilib>:"Add State(s) to Queue__jki_lib_state_machine.vi"("State(s) in (\"\")"=w366) -> ("States Out"=w365:string)  [unwired: 14 in]
      }
      frame "Data: Cleanup" {
        n152 = Unbundle By Name(w368) -> ("Core.Current VI Reference"=w370:refnum<vi>)
        n153 = Close Reference(reference=w370, error in (no error)=w367) -> (error out=w369:errorcluster)
        n154 = call <vilib>:"Add State(s) to Queue__jki_lib_state_machine.vi"("State(s) in (\"\")"=w372) -> ("States Out"=w371:string)  [unwired: 14 in]
      }
      frame "---------- UI ----------" {
        # "Do not put any code in this frame.\n(It is a separator no-op. You can make a copy of this frame to create a new UI frame)"
        n155 = call <vilib>:"Add State(s) to Queue__jki_lib_state_machine.vi"("State(s) in (\"\")"=w376) -> ("States Out"=w375:string)  [unwired: 14 in]
      }
      frame "UI: Stepper Fields Set Enabled" {
        w377 = T9."Enabled" ("Disabled")
        # "Set Stepper Fields state .\n(Usage: \"UI: Stepper Fields Set Enabled >> 'Stepper Number'\")"
        n156 = property on="St1:NewPosition" class="DigNum (strict)"("DisabledEnum"=w377) -> ()  [unwired: 2 in, 2 out]
        n157 = property on="St2:NewPosition" class="DigNum (strict)"("DisabledEnum"=w377) -> ()  [unwired: 2 in, 2 out]
        n158 = property on="St1:Steps" class="DigNum (strict)"("DisabledEnum"=w377) -> ()  [unwired: 2 in, 2 out]
        n159 = property on="St2:Steps" class="DigNum (strict)"("DisabledEnum"=w377) -> ()  [unwired: 2 in, 2 out]
        n160 = property on="St3:NewPosition" class="DigNum (strict)"("DisabledEnum"=w377) -> ()  [unwired: 2 in, 2 out]
        n161 = property on="St3:Steps" class="DigNum (strict)"("DisabledEnum"=w377) -> ()  [unwired: 2 in, 2 out]
        n162 = property on="St:DoSteps" class="Bool (strict)"("DisabledEnum"=w377) -> ()  [unwired: 2 in, 2 out]
        n163 = call <vilib>:"Add State(s) to Queue__jki_lib_state_machine.vi"("State(s) in (\"\")"=w381) -> ("States Out"=w380:string)  [unwired: 14 in]
      }
      frame "UI: Stepper Fields Set Disabled" {
        w382 = T9."Disabled and Grayed Out" ("Disabled")
        # "Set Stepper Fields state .\n(Usage: \"UI: Stepper Fields Set Enabled >> 'Stepper Number'\")"
        n164 = property on="St1:NewPosition" class="DigNum (strict)"("DisabledEnum"=w382) -> ()  [unwired: 2 in, 2 out]
        n165 = property on="St1:Steps" class="DigNum (strict)"("DisabledEnum"=w382) -> ()  [unwired: 2 in, 2 out]
        n166 = property on="St2:NewPosition" class="DigNum (strict)"("DisabledEnum"=w382) -> ()  [unwired: 2 in, 2 out]
        n167 = property on="St2:Steps" class="DigNum (strict)"("DisabledEnum"=w382) -> ()  [unwired: 2 in, 2 out]
        n168 = property on="St3:NewPosition" class="DigNum (strict)"("DisabledEnum"=w382) -> ()  [unwired: 2 in, 2 out]
        n169 = property on="St3:Steps" class="DigNum (strict)"("DisabledEnum"=w382) -> ()  [unwired: 2 in, 2 out]
        n170 = property on="St:DoSteps" class="Bool (strict)"("DisabledEnum"=w382) -> ()  [unwired: 2 in, 2 out]
        n171 = call <vilib>:"Add State(s) to Queue__jki_lib_state_machine.vi"("State(s) in (\"\")"=w386) -> ("States Out"=w385:string)  [unwired: 14 in]
      }
      frame "UI: Initialize" {
        n172 = call <vilib>:"Add State(s) to Queue__jki_lib_state_machine.vi"("State(s) in Front (\"\")"="UI: Stepper Fields Set Enabled" ("State(s) in Front (\"\")"), "State(s) in (\"\")"=w391) -> ("States Out"=w390:string)  [unwired: 13 in]
      }
      frame "UI: Steps to new position" {
        n173 = case shown="\"3\"" w392 {
          frame "1" {
            n174 = local read "St1:Position"() -> (w398:dbl)
            n175 = local read "St1:Steps"() -> (w397:dbl)
            n176 = Add(x=w398, y=w397) -> (x+y=w396:dbl)
            n177 = local write "St1:NewPosition"(w396) -> ()
          }
          frame "2" {
            n178 = local read "St2:Position"() -> (w401:dbl)
            n179 = local read "St2:Steps"() -> (w400:dbl)
            n180 = Add(x=w401, y=w400) -> (x+y=w399:dbl)
            n181 = local write "St2:NewPosition"(w399) -> ()
          }
          frame "3" {
            n182 = local read "St3:Position"() -> (w404:dbl)
            n183 = local read "St3:Steps"() -> (w403:dbl)
            n184 = Add(x=w404, y=w403) -> (x+y=w402:dbl)
            n185 = local write "St3:NewPosition"(w402) -> ()
          }
          frame Default {
          }
        }
      }
      frame "UI: New WL to positions" {
        n186 = local read "WL:WLToStepper1"() -> (w411:dbl[][])
        n187 = local read "WL:WLToStepper2"() -> (w409:dbl[][])
        n188 = local read "WL:WLToStepper3"() -> (w410:dbl[][])
        n189 = property on="WL:NewValue" class="DigNum (strict)"() -> ("Value"=w405:dbl)  [unwired: 2 in, 2 out]
        n190 = call "GetNearestValue.vi"("Value"=w405, "Array"=w411) -> ("Nearest Value"=w408:dbl)  [unwired: 9 in]
        n191 = call "GetNearestValue.vi"("Value"=w405, "Array"=w409) -> ("Nearest Value"=w407:dbl)  [unwired: 9 in]
        n192 = call "GetNearestValue.vi"("Value"=w405, "Array"=w410) -> ("Nearest Value"=w406:dbl)  [unwired: 9 in]
        n193 = property on="St1:NewPosition" class="DigNum (strict)"("Val(Sgnl)"=w408) -> ()  [unwired: 2 in, 2 out]
        n194 = property on="St2:NewPosition" class="DigNum (strict)"("Val(Sgnl)"=w407) -> ()  [unwired: 2 in, 2 out]
        n195 = property on="St3:NewPosition" class="DigNum (strict)"("Val(Sgnl)"=w406) -> ()  [unwired: 2 in, 2 out]
      }
      frame "UI: New position to steps" {
        n196 = case shown="Default" w416 {
          frame Default {
          }
          frame "1" {
            n197 = local read "St1:NewPosition"() -> (w421:dbl)
            n198 = local read "St1:Position"() -> (w420:dbl)
            n199 = Subtract(x=w421, y=w420) -> (x-y=w419:dbl)
            n200 = local write "St1:Steps"(w419) -> ()
          }
          frame "2" {
            n201 = local read "St2:NewPosition"() -> (w424:dbl)
            n202 = local read "St2:Position"() -> (w423:dbl)
            n203 = Subtract(x=w424, y=w423) -> (x-y=w422:dbl)
            n204 = local write "St2:Steps"(w422) -> ()
          }
          frame "3" {
            n205 = local read "St3:NewPosition"() -> (w427:dbl)
            n206 = local read "St3:Position"() -> (w426:dbl)
            n207 = Subtract(x=w427, y=w426) -> (x-y=w425:dbl)
            n208 = local write "St3:Steps"(w425) -> ()
          }
        }
      }
      frame "UI: Cursor Set" {
        # "Set and Unset Cursor Busy.\n(Usage: \"UI: Cursor Set >> Busy|Idle\")"
        n209 = call <vilib>:"Add State(s) to Queue__jki_lib_state_machine.vi"("State(s) in (\"\")"=w431) -> ("States Out"=w430:string)  [unwired: 14 in]
      }
      frame "UI: RefreshLED Set" {
        # "Argument"
        # "Set and Unset RefreshLED.\n(Usage: \"UI: RefreshLED Set >> On|Off\")"
        n210 = case shown="\"Off\", Default" w435 {
          tunnel: [TRUE FALSE] -> w433
          frame "On" {
          }
          frame "Off", Default {
          }
        }
        "App:RefreshLED" <- w433
      }
      frame "UI: Front Panel State" {
        # "Argument"
        # "Set Front Panel Open or Closed\n(Usage: \"UI: Front Panel State >> Open|Close\")"
        n211 = Unbundle By Name(w442) -> ("Core.Current VI Reference"=w441:refnum<vi>)
        n212 = case shown="\"Open\", Default" w440 {
          tunnel: w444 -> [w446 w450]
          tunnel: [w445 w448] -> w443
          tunnel: w441 -> [w447 w449]
          frame "Open", Default {
            n213 = property class="VI" props=["Front Panel.Open"](reference=w447, error in=w446) -> (error out=w445:errorcluster)  [unwired: 2 out]
          }
          frame "Close" {
            n214 = property class="VI" props=["Front Panel.Open"](reference=w449, error in=w450) -> (error out=w448:errorcluster)  [unwired: 2 out]
          }
        }
      }
      frame "---------- Macro ----------" {
        # "Do not put any code in this frame.\n(It is a separator no-op. You can make a copy of this frame to create a new Macro frame)"
        n215 = call <vilib>:"Add State(s) to Queue__jki_lib_state_machine.vi"("State(s) in (\"\")"=w454) -> ("States Out"=w453:string)  [unwired: 14 in]
      }
      frame "Macro: Initialize" {
        w455 = "Data: Initialize\nInitialize Core Data\nUI: Initialize\nUI: Front Panel State >> Open\nData: Load Conversion Files\nData: Read Config\nSteppers: Connect"  # Data: Initialize Initialize Core Data UI: Initialize UI: Front Panel State >> Open Data: Load Conversion Files Data: Read Config Steppers: Connect
        # "Initialization Macro\n(This is called once, when the VI starts)"
        n216 = call <vilib>:"Add State(s) to Queue__jki_lib_state_machine.vi"("State(s) in Front (\"\")"=w455, "State(s) in (\"\")"=w459) -> ("States Out"=w458:string)  [unwired: 13 in]
      }
      frame "Macro: Refresh" {
        n217 = call <vilib>:"Add State(s) to Queue__jki_lib_state_machine.vi"("State(s) in Front (\"\")"="UI: RefreshLED Set >> On\nSteppers: Refresh\nUI: RefreshLED Set >> Off", "State(s) in (\"\")"=w464) -> ("States Out"=w463:string)  [unwired: 13 in]
      }
      frame "Macro: Exit" {
        # "Exit Macro\n(This is called once, when the VI exits)"
        n218 = Unbundle By Name(w471) -> ("Core.Close Panel on Exit?"=w470:bool)
        n219 = Select(t="UI: Front Panel State >> Close", s=w470, f="") -> (s? t:f=w467:string)
        n220 = call <vilib>:"Add State(s) to Queue__jki_lib_state_machine.vi"("State(s) in (\"\")"=w467, "State(s) at Back (\"\")"="Steppers: Disconnect\nData: Cleanup\nExit") -> ("States Out"=w465:string)  [unwired: 13 in]
        n221 = call <vilib>:"Add State(s) to Queue__jki_lib_state_machine.vi"("State(s) in Front (\"\")"=w465, "State(s) in (\"\")"=w474) -> ("States Out"=w473:string)  [unwired: 13 in]
      }
      frame "---------- Steppers ----------" {
        # "Template Separator\n(You can make a copy of, or modify, this frame)"
        n222 = call <vilib>:"Add State(s) to Queue__jki_lib_state_machine.vi"("State(s) in (\"\")"=w478) -> ("States Out"=w477:string)  [unwired: 14 in]
      }
      frame "Steppers: Connect" {
        # "Connect to steppers"
        n223 = call "Send Connect.vi"("error in (no error)"=w481, "Message Enqueuer"=w482) -> ("error out"=w479:errorcluster)  [unwired: 8 in, 1 out]
        n224 = call <vilib>:"Add State(s) to Queue__jki_lib_state_machine.vi"("State(s) in Front (\"\")"="Macro: Refresh\nSteppers: Set position >> 1\nSteppers: Set position >> 2\nSteppers: Set position >> 3" ("State(s) at Back (\"\")"), "State(s) in (\"\")"=w484) -> ("States Out"=w485:string)  [unwired: 13 in]
      }
      frame "Steppers: Disconnect" {
        n225 = call "Send Disconnect.vi"("error in (no error)"=w488, "Message Enqueuer"=w489) -> ("error out"=w487:errorcluster)  [unwired: 8 in, 1 out]
      }
      frame "Steppers: Do steps" {
        n226 = local read "WL:NewValue"() -> (w491:dbl)
        n227 = call "Write Double.vi"("value"=w491, "DataSingleElement in"=refnum<class "DataSingleElement.lvclass"> refnum ("DataSingleElement.lvclass")) -> ("DataSingleElement out"=w492:refnum<class "DataSingleElement.lvclass">)  [unwired: 8 in, 1 out]
        n228 = call "Send Set Parameter.vi"("Parameter"=w492, "Message Enqueuer"=w494) -> ()  [unwired: 8 in, 2 out]
        n229 = call <vilib>:"Add State(s) to Queue__jki_lib_state_machine.vi"("State(s) in (\"\")"=w498) -> ("States Out"=w497:string)  [unwired: 14 in]
      }
      frame "Steppers: Set position" {
        w506 = 0.0
        n230 = case shown="\"1\"" w509 {
          tunnel: [0 ("St3:Steps") w515 w516 w517] -> w501
          frame Default {
          }
          frame "1" {
            n231 = local read "St1:NewPosition"() -> (w515:dbl)
          }
          frame "2" {
            n232 = local read "St2:NewPosition"() -> (w516:dbl)
          }
          frame "3" {
            n233 = local read "St3:NewPosition"() -> (w517:dbl)
          }
        }
        n234 = Decimal String To Number(string=w509, default (0L)=u16 0 ("default (0 I32)")) -> (number=w504:u16)  [unwired: 1 in, 1 out]
        n235 = Decrement(x=w504) -> (x-1=w503:u16)
        n236 = Unbundle By Name(w510) -> ("App:ResourceName"=w499:refnum<visa-resource-name>)
        n237 = Build Array(w506, w506, w506) -> (w505:dbl[])
        n238 = Replace Array Subset(array=w505, new element=w501, index=w503) -> (w500:dbl[])
        n239 = call "SetPosition.vi"("error in (no error)"=w507, "positions"=w500, "VISA Refnum in"=w499) -> ("error out"=w508:errorcluster)  [unwired: 7 in, 1 out]
        n240 = call <vilib>:"Add State(s) to Queue__jki_lib_state_machine.vi"("State(s) in (\"\")"=w513, "State(s) at Back (\"\")"="Data: Write Config" ("State(s) at Back (\"\")")) -> ("States Out"=w512:string)  [unwired: 13 in]
      }
      frame "Steppers: Stop" {
        n241 = Unbundle By Name(w522) -> ("App:ResourceName"=w521:refnum<visa-resource-name>)
        n242 = call "Stop.vi"("error in (no error)"=w520, "VISA Refnum in"=w521) -> ("error out"=w519:errorcluster)  [unwired: 8 in, 1 out]
        n243 = call <vilib>:"Add State(s) to Queue__jki_lib_state_machine.vi"("State(s) in (\"\")"=w524, "State(s) at Back (\"\")"="Data: Write Config" ("State(s) at Back (\"\")")) -> ("States Out"=w523:string)  [unwired: 13 in]
      }
      frame "Steppers: Refresh" {
        n244 = call "Send Refresh Info.vi"("error in (no error)"=w526, "Message Enqueuer"=w527) -> ("error out"=w525:errorcluster)  [unwired: 8 in, 1 out]
        n245 = call <vilib>:"Add State(s) to Queue__jki_lib_state_machine.vi"("State(s) in Front (\"\")"="UI: New position to steps >> 1\nUI: New position to steps >> 2\nUI: New position to steps >> 3\nData: Write Config" ("State(s) at Back (\"\")"), "State(s) in (\"\")"=w530) -> ("States Out"=w529:string)  [unwired: 13 in]
      }
      frame "---------- Utils ---------" {
        # "Template Separator\n(You can make a copy of, or modify, this frame)"
        n246 = call <vilib>:"Add State(s) to Queue__jki_lib_state_machine.vi"("State(s) in (\"\")"=w535) -> ("States Out"=w534:string)  [unwired: 14 in]
      }
      frame "Utils: Wait ms" {
        # "Wait ms >> \"number of ms\""
        n247 = Decimal String To Number(string=w538, default (0L)=u32 0 ("default (0 I32)")) -> (number=w537:u32)  [unwired: 1 in, 1 out]
        n248 = Wait (ms)(milliseconds to wait=w537) -> ()  [unwired: 1 out]
        n249 = call <vilib>:"Add State(s) to Queue__jki_lib_state_machine.vi"("State(s) in (\"\")"=w542) -> ("States Out"=w541:string)  [unwired: 14 in]
      }
    }
  }
  n250 = call-parent "Call Parent Method"("error in"=w10, "Actor in"=w11) -> ("error out"=w9:errorcluster, "Actor out"=w8:refnum<class "Actor.lvclass">)  [unwired: 8 in]
  n251 = call "Send Last Stop Event.vi"("error in (no error)"=w9, "Actor in"=w8) -> ("error out"=→"error out":errorcluster, "Actor  out"=→"Actor  out":refnum<class "Actor.lvclass">)  [unwired: 8 in]
  "Stop" <- FALSE ("Stop")
